vi "Init Tickboxes.vi"(8 "Error In":errorcluster, 11 "Module Data":T1) -> (0 "Error Out":errorcluster)   [LabVIEW 2022 SP3]
doc: "This VI configures the initial state of the three \"Add To ...?\" tickboxes, and the associated string indicators, combo boxes, and captions.\n\nSee \"Design Spreadsheet.xlsx\" for details."
uses:
  Module Data.ctl
  GUI Object Refs (cluster).ctl
  Initial State (enum).ctl
  Input Conditions (cluster).ctl
  DFS Output (cluster).ctl
panel:
  # "Development\nControls or indicators that are useful for development or testing, but which are not outputs of the VI."
  # "Input\nInputs to the VI"
  # "Output\nOutputs of the VI"
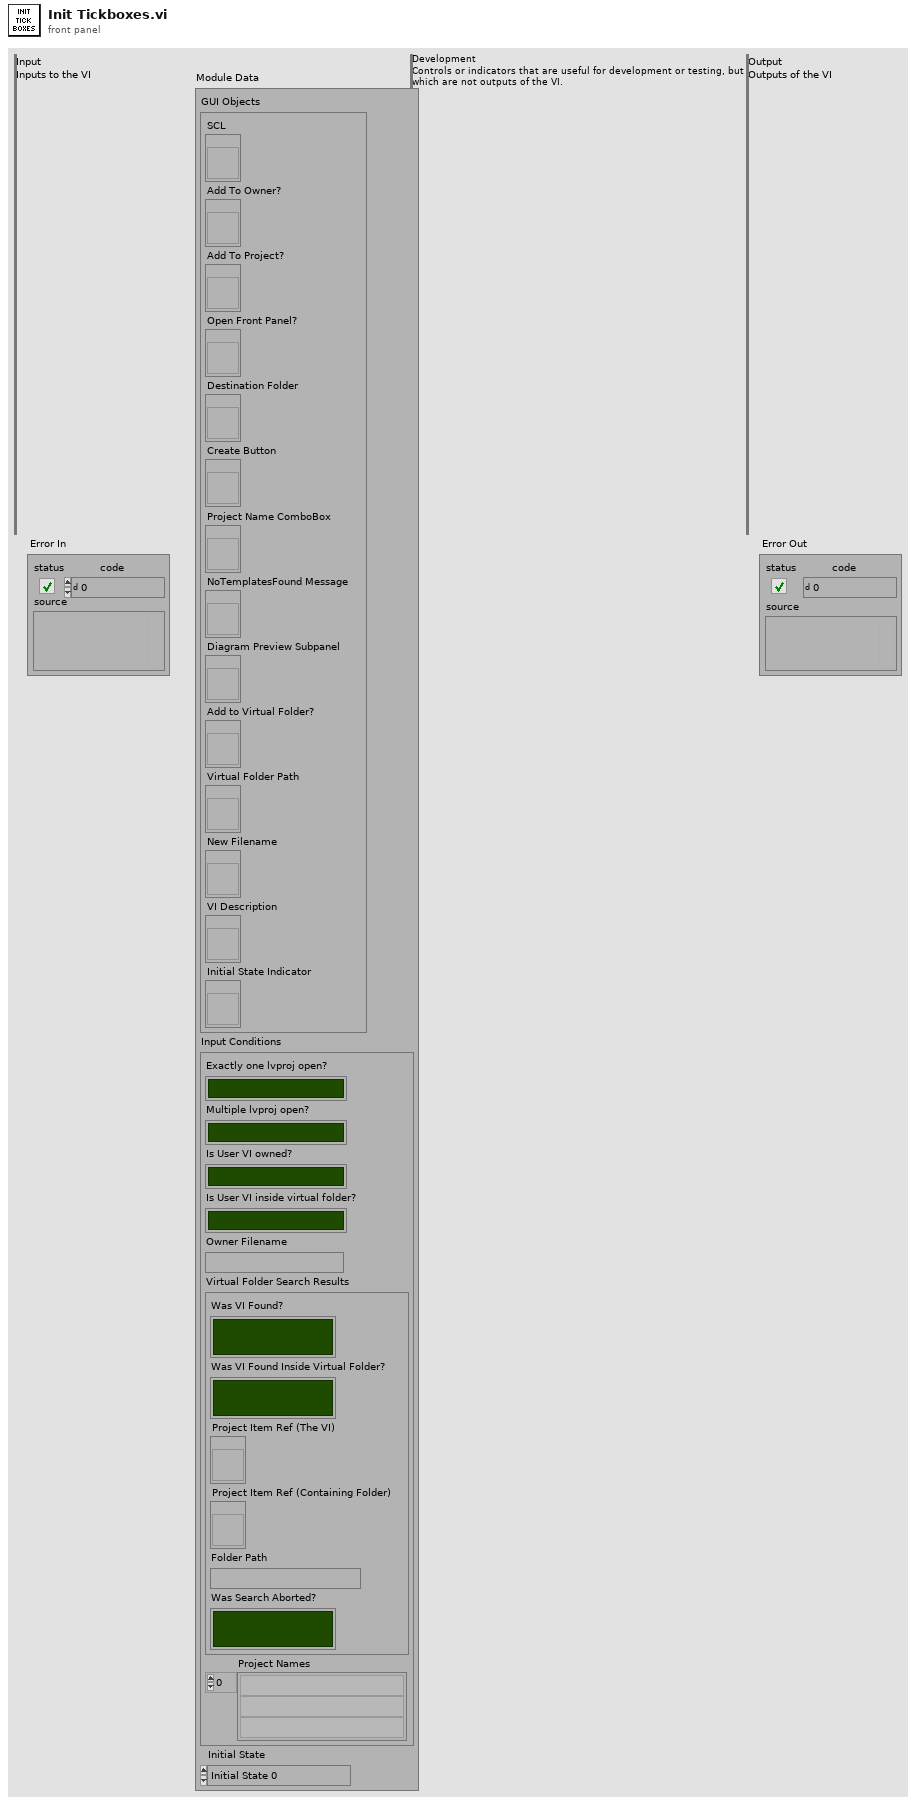
[diagram p1: front panel]
types:
  T1 = typedef "Module Data.ctl" = cluster{"GUI Objects":T2, "Input Conditions":T3, "Initial State":T5}
  T2 = typedef "GUI Object Refs (cluster).ctl" = cluster{"SCL":refnum<vi>, "Add To Owner?":refnum<vi>, "Add To Project?":refnum<vi>, "Open Front Panel?":refnum<vi>, "Destination Folder":refnum<vi>, "Create Button":refnum<vi>, "Project Name ComboBox":refnum<vi>, "NoTemplatesFound Message":refnum<vi>, "Diagram Preview Subpanel":refnum<vi>, "Add to Virtual Folder?":refnum<vi>, "Virtual Folder Path":refnum<vi>, "New Filename":refnum<vi>, "VI Description":refnum<vi>, "Initial State Indicator":refnum<vi>}
  T3 = typedef "Input Conditions (cluster).ctl" = cluster{"Exactly one lvproj open?":bool, "Multiple lvproj open?":bool, "Is User VI owned?":bool, "Is User VI inside virtual folder?":bool, "Owner Filename":string, "Virtual Folder Search Results":T4, "Project Names":string[]}
  T4 = typedef "DFS Output (cluster).ctl" = cluster{"Was VI Found?":bool, "Was VI Found Inside Virtual Folder?":bool, "Project Item Ref (The VI)":refnum<vi>, "Project Item Ref (Containing Folder)":refnum<vi>, "Folder Path":string, "Was Search Aborted?":bool}
  T5 = typedef "Initial State (enum).ctl" = enum16{"Initial State 0", "Initial State 1", "Initial State 2", "Initial State 3", "Initial State 4", "Initial State 5", "Initial State 6", "Initial State 7", "Initial State 8", "Initial State 9", "Initial State 10", "Initial State 11", "Initial State 12", "Initial State 13", "Initial State 14", "Initial State 15"}
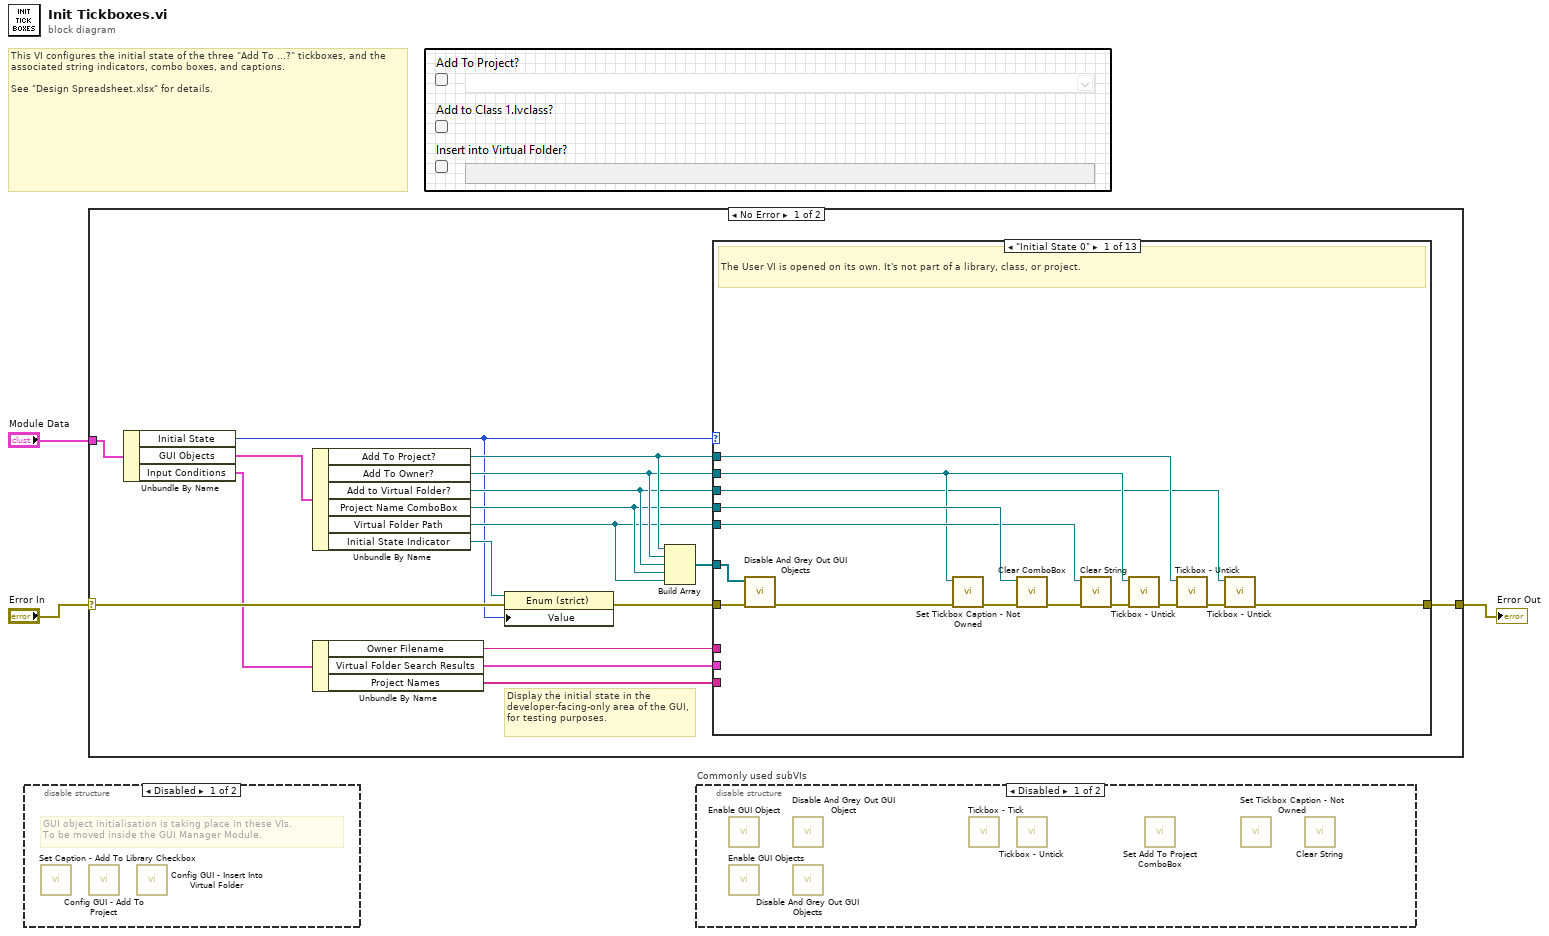
[diagram p0: block diagram]
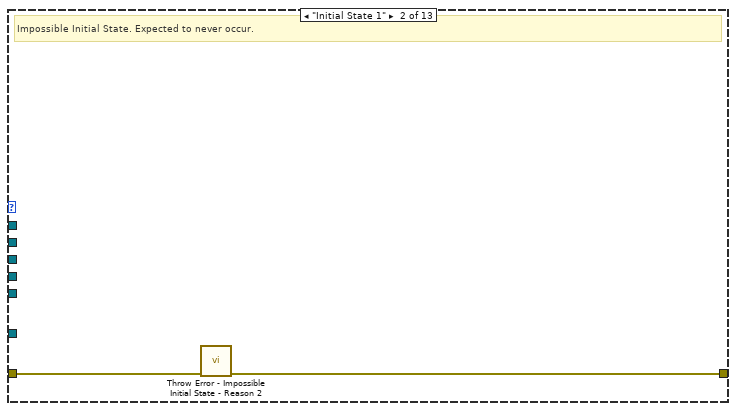
[diagram p4: hidden frame]
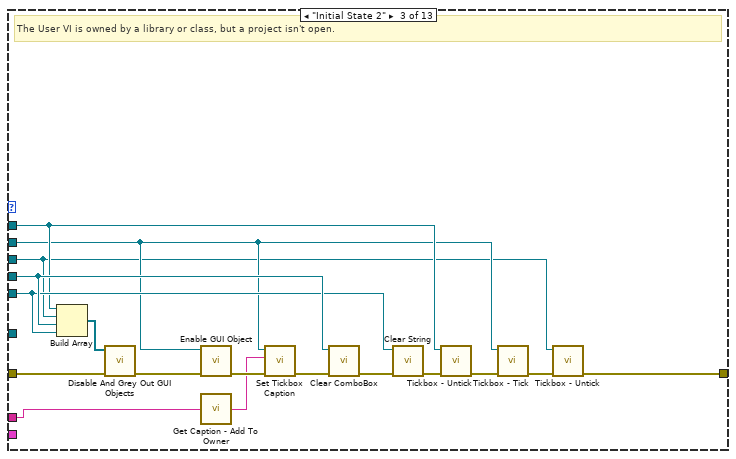
[diagram p5: hidden frame]
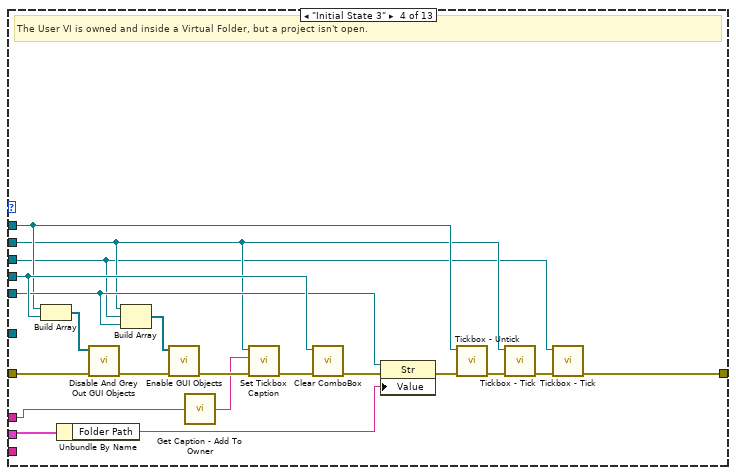
[diagram p6: hidden frame]
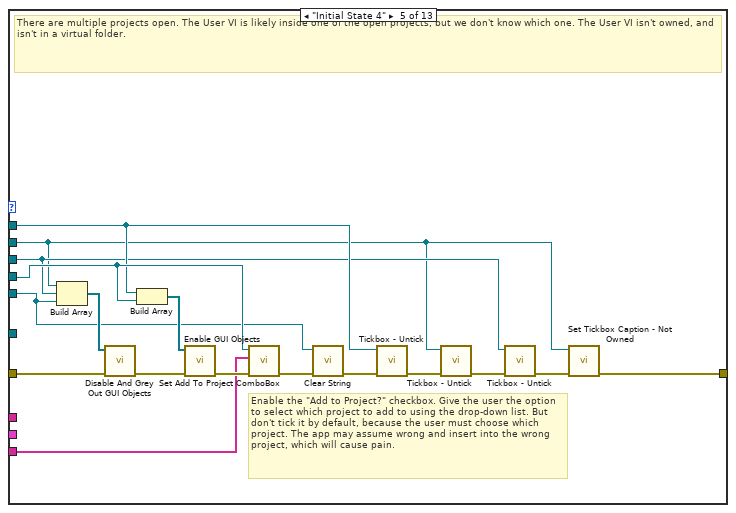
[diagram p7: hidden frame]
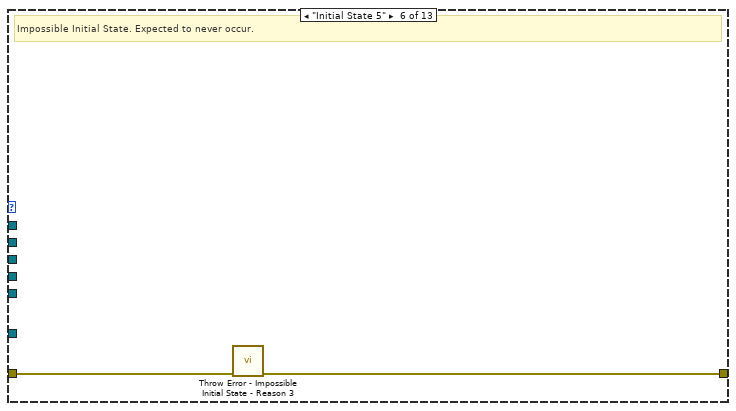
[diagram p8: hidden frame]
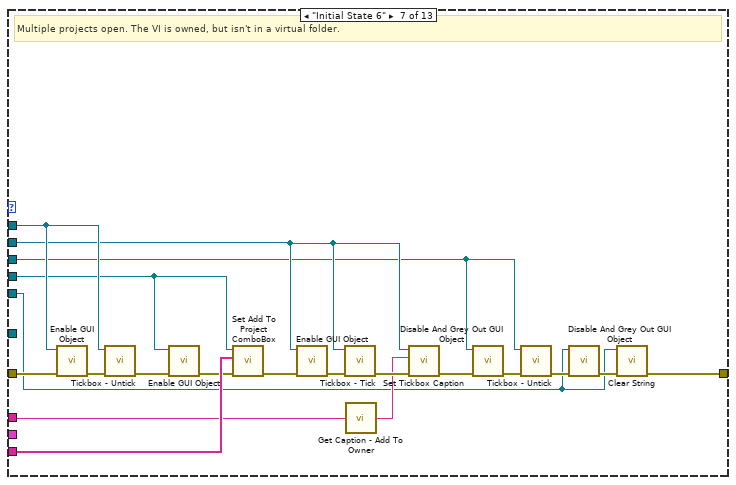
[diagram p9: hidden frame]
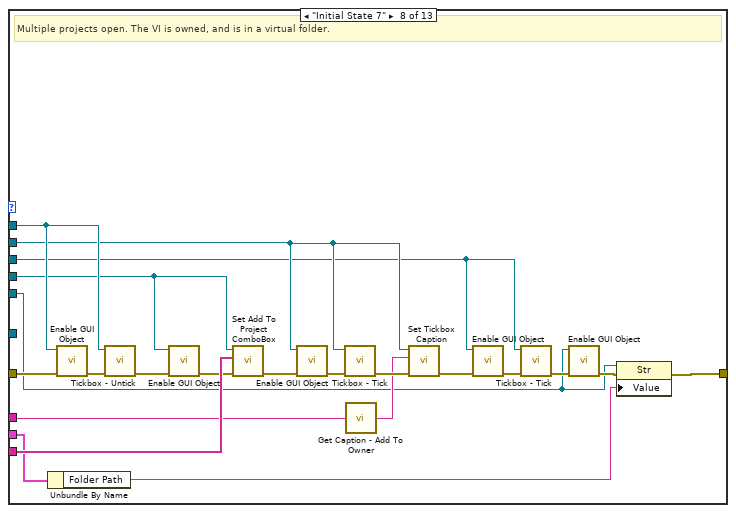
[diagram p10: hidden frame]
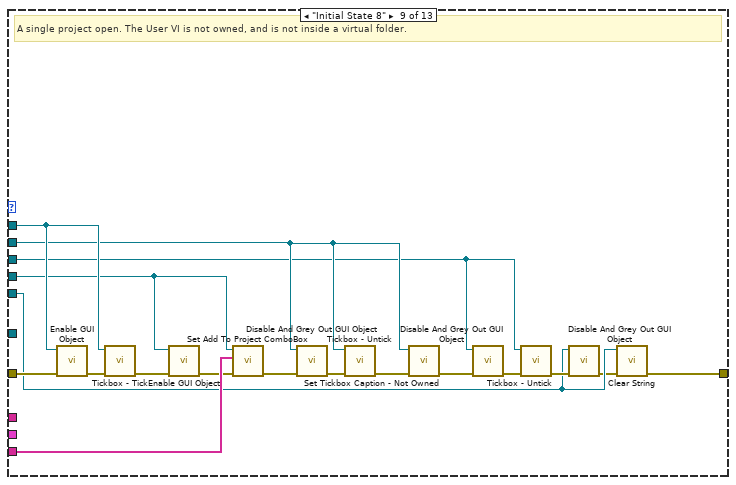
[diagram p11: hidden frame]
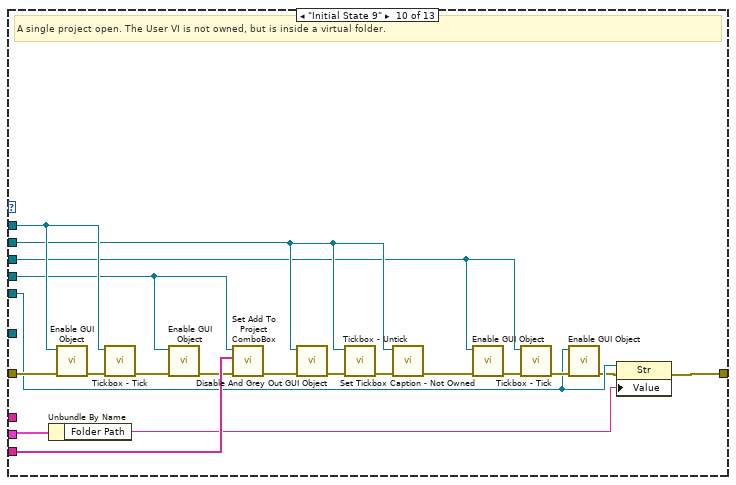
[diagram p12: hidden frame]
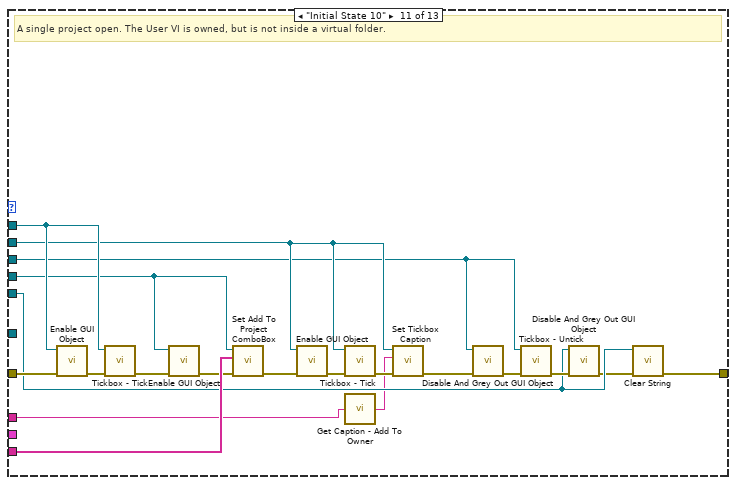
[diagram p13: hidden frame]
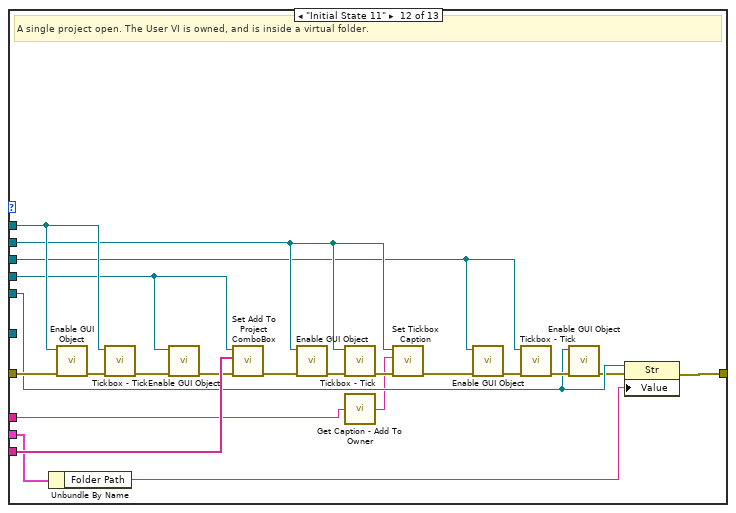
[diagram p14: hidden frame]
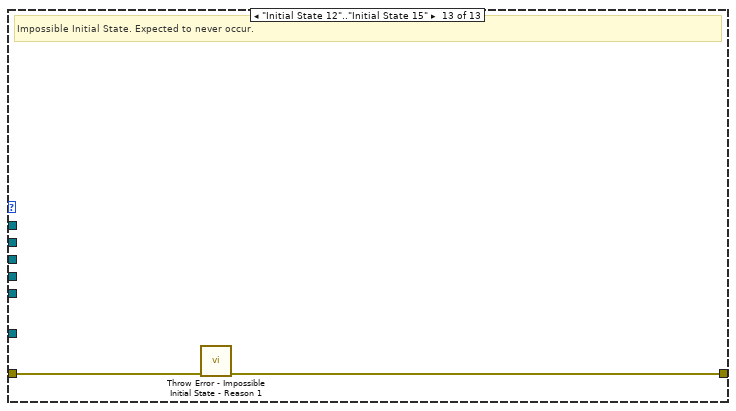
[diagram p15: hidden frame]
diagram:
  # "This VI configures the initial state of the three \"Add To ...?\" tickboxes, and the associated string indicators, combo boxes, and captions.\n\nSee \"Design Spreadsheet.xlsx\" for details."
  n1 = disable-structure shown="Disabled" {
    frame Disabled {
      # "GUI object initialisation is taking place in these VIs.\nTo be moved inside the GUI Manager Module."
      n2 = call "Set Caption - Add To Library Checkbox.vi"() -> ()  [unwired: 11 in, 1 out]
      n3 = call "Config GUI - Add To Project.vi"() -> ()  [unwired: 7 in, 5 out]
      n4 = call "Config GUI - Insert Into Virtual Folder.vi"() -> ()  [unwired: 11 in, 1 out]
    }
    frame Enabled {
    }
  }
  n5 = case shown="No Error" "Error In" {
    selector: "Error In" -> [w20 w217]
    tunnel: [w18 w217] -> w2
    tunnel: "Module Data" -> [w19 _]
    frame No Error {
      # "Display the initial state in the developer-facing-only area of the GUI, for testing purposes."
      n6 = Unbundle By Name(w19) -> ("Initial State"=w4:T5, "GUI Objects"=w17:T2, "Input Conditions"=w10:T3)
      n7 = Unbundle By Name(w17) -> ("Add To Project?"=w16:refnum<vi>, "Add To Owner?"=w15:refnum<vi>, "Add to Virtual Folder?"=w14:refnum<vi>, "Project Name ComboBox"=w13:refnum<vi>, "Virtual Folder Path"=w12:refnum<vi>, "Initial State Indicator"=w5:refnum<vi>)
      n8 = Unbundle By Name(w10) -> ("Owner Filename"=w9:string, "Virtual Folder Search Results"=w8:T4, "Project Names"=w7:string[])
      n9 = property class="Enum (strict)"(reference=w5, error in=w20, "Value"=w4) -> (error out=w6:errorcluster)  [unwired: 1 out]
      n10 = Build Array(w16, w15, w14, w13, w12) -> (w11:refnum<vi>[])
      n11 = case shown="\"Initial State 0\"" w4 {
        tunnel: w6 -> [w33 w36 w53 w73 w90 w92 w112 w134 w152 w172 w192 w214 w216]
        tunnel: [w24 w35 w38 w56 w75 w91 w94 w116 w137 w157 w177 w199 w215] -> w18
        tunnel: w16 -> [w22 _ w41 w58 w78 _ w110 w132 w150 w170 w190 w212 _]
        tunnel: w15 -> [w23 _ w39 w55 w74 _ w101 w123 w142 w162 w182 w204 _]
        tunnel: w14 -> [w21 _ w37 w54 w77 _ w97 w119 w139 w159 w179 w201 _]
        tunnel: w13 -> [w29 _ w44 w65 w85 _ w106 w128 w146 w166 w186 w208 _]
        tunnel: w12 -> [w28 _ w43 w62 w76 _ w93 w115 w136 w156 w176 w198 _]
        tunnel: w11 -> [w32 _ _ _ _ _ _ _ _ _ _ _ _]
        tunnel: w9 -> [_ _ w45 w66 _ _ w100 w122 _ _ w174 w196 _]
        tunnel: w8 -> [_ _ _ w61 _ _ _ w114 _ w154 _ w194 _]
        tunnel: w7 -> [_ _ _ _ w84 _ w109 w131 w149 w169 w189 w211 _]
        frame "Initial State 0" {
          # "The User VI is opened on its own. It's not part of a library, class, or project."
          n12 = call "Disable And Grey Out GUI Objects.vi"("Error In"=w33, "GUI Object Refs"=w32) -> ("Error Out"=w34:errorcluster)  [unwired: 9 in]
          n13 = call "Set Tickbox Caption - Not Owned.vi"("Error In"=w34, "Tickbox Ref"=w23) -> ("Error Out"=w31:errorcluster)  [unwired: 9 in]
          n14 = call "Clear ComboBox.vi"("Error In"=w31, "ComboBox Ref"=w29) -> ("Error Out"=w30:errorcluster)  [unwired: 9 in]
          n15 = call "Clear String.vi"("Error In"=w30, "String Ref"=w28) -> ("Error Out"=w27:errorcluster)  [unwired: 9 in]
          n16 = call "Tickbox - Untick.vi"("Error In"=w27, "Tickbox Ref"=w23) -> ("Error Out"=w26:errorcluster)  [unwired: 9 in]
          n17 = call "Tickbox - Untick.vi"("Error In"=w26, "Tickbox Ref"=w22) -> ("Error Out"=w25:errorcluster)  [unwired: 9 in]
          n18 = call "Tickbox - Untick.vi"("Error In"=w25, "Tickbox Ref"=w21) -> ("Error Out"=w24:errorcluster)  [unwired: 9 in]
        }
        frame "Initial State 1" {
          # "Impossible Initial State. Expected to never occur."
          n19 = call "Throw Error - Impossible Initial State - Reason 2.vi"("error in"=w36) -> ("error out"=w35:errorcluster)  [unwired: 10 in]
        }
        frame "Initial State 2" {
          # "The User VI is owned by a library or class, but a project isn't open."
          n20 = Build Array(w41, w37, w44, w43) -> (w52:refnum<vi>[])
          n21 = call "Disable And Grey Out GUI Objects.vi"("Error In"=w53, "GUI Object Refs"=w52) -> ("Error Out"=w48:errorcluster)  [unwired: 9 in]
          n22 = call "Enable GUI Object.vi"("Error In"=w48, "GUI Object Ref"=w39) -> ("Error Out"=w47:errorcluster)  [unwired: 9 in]
          n23 = call "Get Caption - Add To Owner.vi"("Owner Filename (incl. file extension)"=w45) -> ("\"Add To Owner\" caption"=w46:string)
          n24 = call "Set Tickbox Caption.vi"("Error In"=w47, "Caption"=w46, "Tickbox Ref"=w39) -> ("Error Out"=w51:errorcluster)  [unwired: 8 in]
          n25 = call "Clear ComboBox.vi"("Error In"=w51, "ComboBox Ref"=w44) -> ("Error Out"=w50:errorcluster)  [unwired: 9 in]
          n26 = call "Clear String.vi"("Error In"=w50, "String Ref"=w43) -> ("Error Out"=w49:errorcluster)  [unwired: 9 in]
          n27 = call "Tickbox - Untick.vi"("Error In"=w49, "Tickbox Ref"=w41) -> ("Error Out"=w42:errorcluster)  [unwired: 9 in]
          n28 = call "Tickbox - Tick.vi"("Error In"=w42, "Tickbox Ref"=w39) -> ("Error Out"=w40:errorcluster)  [unwired: 9 in]
          n29 = call "Tickbox - Untick.vi"("Error In"=w40, "Tickbox Ref"=w37) -> ("Error Out"=w38:errorcluster)  [unwired: 9 in]
        }
        frame "Initial State 3" {
          # "The User VI is owned and inside a Virtual Folder, but a project isn't open."
          n30 = Build Array(w58, w65) -> (w72:refnum<vi>[])
          n31 = Unbundle By Name(w61) -> ("Folder Path"=w60:string)
          n32 = call "Disable And Grey Out GUI Objects.vi"("Error In"=w73, "GUI Object Refs"=w72) -> ("Error Out"=w69:errorcluster)  [unwired: 9 in]
          n33 = Build Array(w55, w54, w62) -> (w64:refnum<vi>[])
          n34 = call "Enable GUI Objects.vi"("Error In"=w69, "GUI Object Refs"=w64) -> ("Error Out"=w68:errorcluster)  [unwired: 9 in]
          n35 = call "Get Caption - Add To Owner.vi"("Owner Filename (incl. file extension)"=w66) -> ("\"Add To Owner\" caption"=w67:string)
          n36 = call "Set Tickbox Caption.vi"("Error In"=w68, "Caption"=w67, "Tickbox Ref"=w55) -> ("Error Out"=w71:errorcluster)  [unwired: 8 in]
          n37 = call "Clear ComboBox.vi"("Error In"=w71, "ComboBox Ref"=w65) -> ("Error Out"=w70:errorcluster)  [unwired: 9 in]
          n38 = property class="Str"(reference=w62, error in=w70, "Value"=w60) -> (error out=w63:errorcluster)  [unwired: 1 out]
          n39 = call "Tickbox - Untick.vi"("Error In"=w63, "Tickbox Ref"=w58) -> ("Error Out"=w59:errorcluster)  [unwired: 9 in]
          n40 = call "Tickbox - Tick.vi"("Error In"=w59, "Tickbox Ref"=w55) -> ("Error Out"=w57:errorcluster)  [unwired: 9 in]
          n41 = call "Tickbox - Tick.vi"("Error In"=w57, "Tickbox Ref"=w54) -> ("Error Out"=w56:errorcluster)  [unwired: 9 in]
        }
        frame "Initial State 4" {
          # "Enable the \"Add to Project?\" checkbox. Give the user the option to select which project to add to using the drop-down list. But don't tick it by default, because the user must choose which project. The app may assume wrong and insert into the wrong project, which will cause pain."
          # "There are multiple projects open. The User VI is likely inside one of the open projects, but we don't know which one. The User VI isn't owned, and isn't in a virtual folder."
          n42 = Build Array(w74, w77, w76) -> (w88:refnum<vi>[])
          n43 = call "Disable And Grey Out GUI Objects.vi"("Error In"=w90, "GUI Object Refs"=w88) -> ("Error Out"=w89:errorcluster)  [unwired: 9 in]
          n44 = Build Array(w78, w85) -> (w87:refnum<vi>[])
          n45 = call "Enable GUI Objects.vi"("Error In"=w89, "GUI Object Refs"=w87) -> ("Error Out"=w86:errorcluster)  [unwired: 9 in]
          n46 = call "Set Add To Project ComboBox.vi"("Error In"=w86, "Project Names"=w84, "Project Name ComboBox Ref"=w85) -> ("Error Out"=w83:errorcluster)  [unwired: 8 in]
          n47 = call "Clear String.vi"("Error In"=w83, "String Ref"=w76) -> ("Error Out"=w82:errorcluster)  [unwired: 9 in]
          n48 = call "Tickbox - Untick.vi"("Error In"=w82, "Tickbox Ref"=w78) -> ("Error Out"=w81:errorcluster)  [unwired: 9 in]
          n49 = call "Tickbox - Untick.vi"("Error In"=w81, "Tickbox Ref"=w74) -> ("Error Out"=w80:errorcluster)  [unwired: 9 in]
          n50 = call "Tickbox - Untick.vi"("Error In"=w80, "Tickbox Ref"=w77) -> ("Error Out"=w79:errorcluster)  [unwired: 9 in]
          n51 = call "Set Tickbox Caption - Not Owned.vi"("Error In"=w79, "Tickbox Ref"=w74) -> ("Error Out"=w75:errorcluster)  [unwired: 9 in]
        }
        frame "Initial State 5" {
          # "Impossible Initial State. Expected to never occur."
          n52 = call "Throw Error - Impossible Initial State - Reason 3.vi"("error in"=w92) -> ("error out"=w91:errorcluster)  [unwired: 10 in]
        }
        frame "Initial State 6" {
          # "Multiple projects open. The VI is owned, but isn't in a virtual folder."
          n53 = call "Enable GUI Object.vi"("Error In"=w112, "GUI Object Ref"=w110) -> ("Error Out"=w111:errorcluster)  [unwired: 9 in]
          n54 = call "Tickbox - Untick.vi"("Error In"=w111, "Tickbox Ref"=w110) -> ("Error Out"=w108:errorcluster)  [unwired: 9 in]
          n55 = call "Enable GUI Object.vi"("Error In"=w108, "GUI Object Ref"=w106) -> ("Error Out"=w107:errorcluster)  [unwired: 9 in]
          n56 = call "Set Add To Project ComboBox.vi"("Error In"=w107, "Project Names"=w109, "Project Name ComboBox Ref"=w106) -> ("Error Out"=w105:errorcluster)  [unwired: 8 in]
          n57 = call "Enable GUI Object.vi"("Error In"=w105, "GUI Object Ref"=w101) -> ("Error Out"=w104:errorcluster)  [unwired: 9 in]
          n58 = call "Tickbox - Tick.vi"("Error In"=w104, "Tickbox Ref"=w101) -> ("Error Out"=w103:errorcluster)  [unwired: 9 in]
          n59 = call "Get Caption - Add To Owner.vi"("Owner Filename (incl. file extension)"=w100) -> ("\"Add To Owner\" caption"=w102:string)
          n60 = call "Set Tickbox Caption.vi"("Error In"=w103, "Caption"=w102, "Tickbox Ref"=w101) -> ("Error Out"=w99:errorcluster)  [unwired: 8 in]
          n61 = call "Disable And Grey Out GUI Object.vi"("Error In"=w99, "GUI Object Ref"=w97) -> ("Error Out"=w98:errorcluster)  [unwired: 9 in]
          n62 = call "Tickbox - Untick.vi"("Error In"=w98, "Tickbox Ref"=w97) -> ("Error Out"=w96:errorcluster)  [unwired: 9 in]
          n63 = call "Disable And Grey Out GUI Object.vi"("Error In"=w96, "GUI Object Ref"=w93) -> ("Error Out"=w95:errorcluster)  [unwired: 9 in]
          n64 = call "Clear String.vi"("Error In"=w95, "String Ref"=w93) -> ("Error Out"=w94:errorcluster)  [unwired: 9 in]
        }
        frame "Initial State 7" {
          # "Multiple projects open. The VI is owned, and is in a virtual folder."
          n65 = Unbundle By Name(w114) -> ("Folder Path"=w113:string)
          n66 = call "Enable GUI Object.vi"("Error In"=w134, "GUI Object Ref"=w132) -> ("Error Out"=w133:errorcluster)  [unwired: 9 in]
          n67 = call "Tickbox - Untick.vi"("Error In"=w133, "Tickbox Ref"=w132) -> ("Error Out"=w130:errorcluster)  [unwired: 9 in]
          n68 = call "Enable GUI Object.vi"("Error In"=w130, "GUI Object Ref"=w128) -> ("Error Out"=w129:errorcluster)  [unwired: 9 in]
          n69 = call "Set Add To Project ComboBox.vi"("Error In"=w129, "Project Names"=w131, "Project Name ComboBox Ref"=w128) -> ("Error Out"=w127:errorcluster)  [unwired: 8 in]
          n70 = call "Enable GUI Object.vi"("Error In"=w127, "GUI Object Ref"=w123) -> ("Error Out"=w126:errorcluster)  [unwired: 9 in]
          n71 = call "Tickbox - Tick.vi"("Error In"=w126, "Tickbox Ref"=w123) -> ("Error Out"=w125:errorcluster)  [unwired: 9 in]
          n72 = call "Get Caption - Add To Owner.vi"("Owner Filename (incl. file extension)"=w122) -> ("\"Add To Owner\" caption"=w124:string)
          n73 = call "Set Tickbox Caption.vi"("Error In"=w125, "Caption"=w124, "Tickbox Ref"=w123) -> ("Error Out"=w121:errorcluster)  [unwired: 8 in]
          n74 = call "Enable GUI Object.vi"("Error In"=w121, "GUI Object Ref"=w119) -> ("Error Out"=w120:errorcluster)  [unwired: 9 in]
          n75 = call "Tickbox - Tick.vi"("Error In"=w120, "Tickbox Ref"=w119) -> ("Error Out"=w118:errorcluster)  [unwired: 9 in]
          n76 = call "Enable GUI Object.vi"("Error In"=w118, "GUI Object Ref"=w115) -> ("Error Out"=w117:errorcluster)  [unwired: 9 in]
          n77 = property class="Str"(reference=w115, error in=w117, "Value"=w113) -> (error out=w116:errorcluster)  [unwired: 1 out]
        }
        frame "Initial State 8" {
          # "A single project open. The User VI is not owned, and is not inside a virtual folder."
          n78 = call "Enable GUI Object.vi"("Error In"=w152, "GUI Object Ref"=w150) -> ("Error Out"=w151:errorcluster)  [unwired: 9 in]
          n79 = call "Tickbox - Tick.vi"("Error In"=w151, "Tickbox Ref"=w150) -> ("Error Out"=w148:errorcluster)  [unwired: 9 in]
          n80 = call "Enable GUI Object.vi"("Error In"=w148, "GUI Object Ref"=w146) -> ("Error Out"=w147:errorcluster)  [unwired: 9 in]
          n81 = call "Set Add To Project ComboBox.vi"("Error In"=w147, "Project Names"=w149, "Project Name ComboBox Ref"=w146) -> ("Error Out"=w145:errorcluster)  [unwired: 8 in]
          n82 = call "Disable And Grey Out GUI Object.vi"("Error In"=w145, "GUI Object Ref"=w142) -> ("Error Out"=w144:errorcluster)  [unwired: 9 in]
          n83 = call "Tickbox - Untick.vi"("Error In"=w144, "Tickbox Ref"=w142) -> ("Error Out"=w143:errorcluster)  [unwired: 9 in]
          n84 = call "Set Tickbox Caption - Not Owned.vi"("Error In"=w143, "Tickbox Ref"=w142) -> ("Error Out"=w141:errorcluster)  [unwired: 9 in]
          n85 = call "Disable And Grey Out GUI Object.vi"("Error In"=w141, "GUI Object Ref"=w139) -> ("Error Out"=w140:errorcluster)  [unwired: 9 in]
          n86 = call "Tickbox - Untick.vi"("Error In"=w140, "Tickbox Ref"=w139) -> ("Error Out"=w138:errorcluster)  [unwired: 9 in]
          n87 = call "Disable And Grey Out GUI Object.vi"("Error In"=w138, "GUI Object Ref"=w136) -> ("Error Out"=w135:errorcluster)  [unwired: 9 in]
          n88 = call "Clear String.vi"("Error In"=w135, "String Ref"=w136) -> ("Error Out"=w137:errorcluster)  [unwired: 9 in]
        }
        frame "Initial State 9" {
          # "A single project open. The User VI is not owned, but is inside a virtual folder."
          n89 = Unbundle By Name(w154) -> ("Folder Path"=w153:string)
          n90 = call "Enable GUI Object.vi"("Error In"=w172, "GUI Object Ref"=w170) -> ("Error Out"=w171:errorcluster)  [unwired: 9 in]
          n91 = call "Tickbox - Tick.vi"("Error In"=w171, "Tickbox Ref"=w170) -> ("Error Out"=w168:errorcluster)  [unwired: 9 in]
          n92 = call "Enable GUI Object.vi"("Error In"=w168, "GUI Object Ref"=w166) -> ("Error Out"=w167:errorcluster)  [unwired: 9 in]
          n93 = call "Set Add To Project ComboBox.vi"("Error In"=w167, "Project Names"=w169, "Project Name ComboBox Ref"=w166) -> ("Error Out"=w165:errorcluster)  [unwired: 8 in]
          n94 = call "Disable And Grey Out GUI Object.vi"("Error In"=w165, "GUI Object Ref"=w162) -> ("Error Out"=w164:errorcluster)  [unwired: 9 in]
          n95 = call "Tickbox - Untick.vi"("Error In"=w164, "Tickbox Ref"=w162) -> ("Error Out"=w163:errorcluster)  [unwired: 9 in]
          n96 = call "Set Tickbox Caption - Not Owned.vi"("Error In"=w163, "Tickbox Ref"=w162) -> ("Error Out"=w161:errorcluster)  [unwired: 9 in]
          n97 = call "Enable GUI Object.vi"("Error In"=w161, "GUI Object Ref"=w159) -> ("Error Out"=w160:errorcluster)  [unwired: 9 in]
          n98 = call "Tickbox - Tick.vi"("Error In"=w160, "Tickbox Ref"=w159) -> ("Error Out"=w158:errorcluster)  [unwired: 9 in]
          n99 = call "Enable GUI Object.vi"("Error In"=w158, "GUI Object Ref"=w156) -> ("Error Out"=w155:errorcluster)  [unwired: 9 in]
          n100 = property class="Str"(reference=w156, error in=w155, "Value"=w153) -> (error out=w157:errorcluster)  [unwired: 1 out]
        }
        frame "Initial State 10" {
          # "A single project open. The User VI is owned, but is not inside a virtual folder."
          n101 = call "Enable GUI Object.vi"("Error In"=w192, "GUI Object Ref"=w190) -> ("Error Out"=w191:errorcluster)  [unwired: 9 in]
          n102 = call "Tickbox - Tick.vi"("Error In"=w191, "Tickbox Ref"=w190) -> ("Error Out"=w188:errorcluster)  [unwired: 9 in]
          n103 = call "Enable GUI Object.vi"("Error In"=w188, "GUI Object Ref"=w186) -> ("Error Out"=w187:errorcluster)  [unwired: 9 in]
          n104 = call "Set Add To Project ComboBox.vi"("Error In"=w187, "Project Names"=w189, "Project Name ComboBox Ref"=w186) -> ("Error Out"=w185:errorcluster)  [unwired: 8 in]
          n105 = call "Enable GUI Object.vi"("Error In"=w185, "GUI Object Ref"=w182) -> ("Error Out"=w184:errorcluster)  [unwired: 9 in]
          n106 = call "Tickbox - Tick.vi"("Error In"=w184, "Tickbox Ref"=w182) -> ("Error Out"=w183:errorcluster)  [unwired: 9 in]
          n107 = call "Get Caption - Add To Owner.vi"("Owner Filename (incl. file extension)"=w174) -> ("\"Add To Owner\" caption"=w175:string)
          n108 = call "Set Tickbox Caption.vi"("Error In"=w183, "Caption"=w175, "Tickbox Ref"=w182) -> ("Error Out"=w181:errorcluster)  [unwired: 8 in]
          n109 = call "Disable And Grey Out GUI Object.vi"("Error In"=w181, "GUI Object Ref"=w179) -> ("Error Out"=w180:errorcluster)  [unwired: 9 in]
          n110 = call "Tickbox - Untick.vi"("Error In"=w180, "Tickbox Ref"=w179) -> ("Error Out"=w178:errorcluster)  [unwired: 9 in]
          n111 = call "Disable And Grey Out GUI Object.vi"("Error In"=w178, "GUI Object Ref"=w176) -> ("Error Out"=w173:errorcluster)  [unwired: 9 in]
          n112 = call "Clear String.vi"("Error In"=w173, "String Ref"=w176) -> ("Error Out"=w177:errorcluster)  [unwired: 9 in]
        }
        frame "Initial State 11" {
          # "A single project open. The User VI is owned, and is inside a virtual folder."
          n113 = Unbundle By Name(w194) -> ("Folder Path"=w193:string)
          n114 = call "Enable GUI Object.vi"("Error In"=w214, "GUI Object Ref"=w212) -> ("Error Out"=w213:errorcluster)  [unwired: 9 in]
          n115 = call "Tickbox - Tick.vi"("Error In"=w213, "Tickbox Ref"=w212) -> ("Error Out"=w210:errorcluster)  [unwired: 9 in]
          n116 = call "Enable GUI Object.vi"("Error In"=w210, "GUI Object Ref"=w208) -> ("Error Out"=w209:errorcluster)  [unwired: 9 in]
          n117 = call "Set Add To Project ComboBox.vi"("Error In"=w209, "Project Names"=w211, "Project Name ComboBox Ref"=w208) -> ("Error Out"=w207:errorcluster)  [unwired: 8 in]
          n118 = call "Enable GUI Object.vi"("Error In"=w207, "GUI Object Ref"=w204) -> ("Error Out"=w206:errorcluster)  [unwired: 9 in]
          n119 = call "Tickbox - Tick.vi"("Error In"=w206, "Tickbox Ref"=w204) -> ("Error Out"=w205:errorcluster)  [unwired: 9 in]
          n120 = call "Get Caption - Add To Owner.vi"("Owner Filename (incl. file extension)"=w196) -> ("\"Add To Owner\" caption"=w197:string)
          n121 = call "Set Tickbox Caption.vi"("Error In"=w205, "Caption"=w197, "Tickbox Ref"=w204) -> ("Error Out"=w203:errorcluster)  [unwired: 8 in]
          n122 = call "Enable GUI Object.vi"("Error In"=w203, "GUI Object Ref"=w201) -> ("Error Out"=w202:errorcluster)  [unwired: 9 in]
          n123 = call "Tickbox - Tick.vi"("Error In"=w202, "Tickbox Ref"=w201) -> ("Error Out"=w200:errorcluster)  [unwired: 9 in]
          n124 = call "Enable GUI Object.vi"("Error In"=w200, "GUI Object Ref"=w198) -> ("Error Out"=w195:errorcluster)  [unwired: 9 in]
          n125 = property class="Str"(reference=w198, error in=w195, "Value"=w193) -> (error out=w199:errorcluster)  [unwired: 1 out]
        }
        frame "Initial State 12".."Initial State 15" {
          # "Impossible Initial State. Expected to never occur."
          n126 = call "Throw Error - Impossible Initial State - Reason 1.vi"("error in"=w216) -> ("error out"=w215:errorcluster)  [unwired: 10 in]
        }
      }
    }
    frame Error {
    }
  }
  "Error Out" <- w2
  n127 = disable-structure "Commonly used subVIs" shown="Disabled" {
    frame Disabled {
      n128 = call "Enable GUI Object.vi"() -> ()  [unwired: 11 in, 1 out]
      n129 = call "Enable GUI Objects.vi"() -> ()  [unwired: 11 in, 1 out]
      n130 = call "Disable And Grey Out GUI Object.vi"() -> ()  [unwired: 11 in, 1 out]
      n131 = call "Disable And Grey Out GUI Objects.vi"() -> ()  [unwired: 11 in, 1 out]
      n132 = call "Tickbox - Tick.vi"() -> ()  [unwired: 11 in, 1 out]
      n133 = call "Tickbox - Untick.vi"() -> ()  [unwired: 11 in, 1 out]
      n134 = call "Set Add To Project ComboBox.vi"() -> ()  [unwired: 11 in, 1 out]
      n135 = call "Set Tickbox Caption - Not Owned.vi"() -> ()  [unwired: 11 in, 1 out]
      n136 = call "Clear String.vi"() -> ()  [unwired: 11 in, 1 out]
    }
    frame Enabled {
    }
  }
